vi "AlazarSampling.vi"(9 "Time Out (s)":dbl, 10 "Sampling (Hz)":dbl, 11 "DeviceIn":i32) -> (0 "Return Code":u32, 3 "DeviceOut":i32)   [LabVIEW 2022 SP3]
doc: "_____AlazarTech, Scope_____\n\nConfigure the capture clock circuitry."
uses:
  C:/AlazarTech/ATS-VI/6.2.0/ATS_ctl/Device_Ctrl.ctl
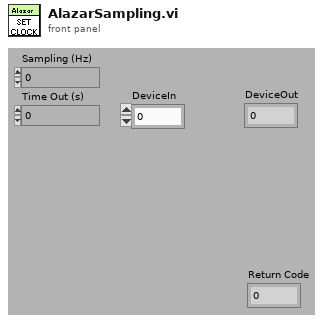
[diagram p1: front panel]
types:
  T1 = typedef "Device_Ctrl.ctl" = enum16{"Status", "About", "Arm", "ForceTrig", "Abort", "Initialize", "Init (NoPreset)", "Info", "Close", "Calibrate", "SetManually", "LED_ON", "LED_OFF"}
  T2 = typedef "Device_Info.ctl" = cluster{"Handle":u32, "Board":string, "CPLD":string, "MemorySize":u32, "SampleSize":u8, "ID":i32, "High_Memory":bool, "Chan/Board":u8}
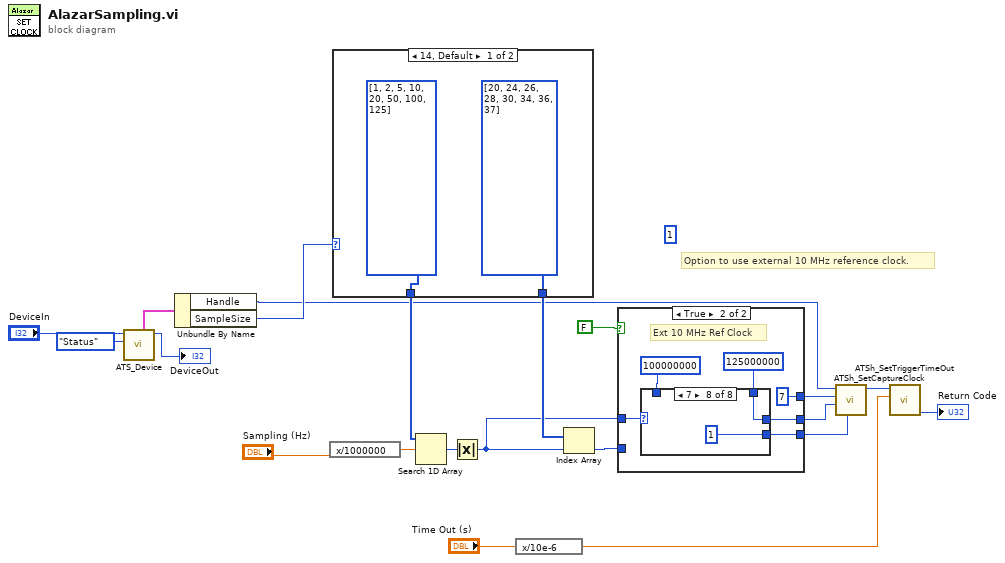
[diagram p0: block diagram]
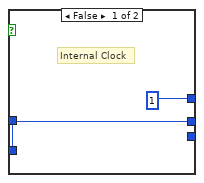
[diagram p2: hidden frame]
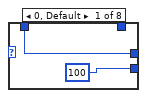
[diagram p3: hidden frame]
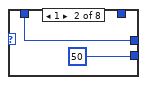
[diagram p4: hidden frame]
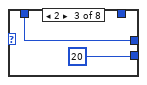
[diagram p5: hidden frame]
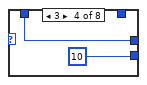
[diagram p6: hidden frame]
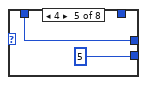
[diagram p7: hidden frame]
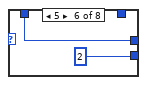
[diagram p8: hidden frame]
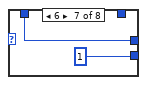
[diagram p9: hidden frame]
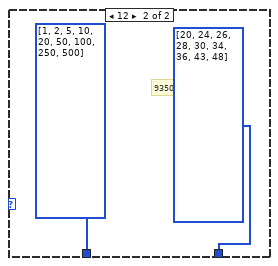
[diagram p10: hidden frame]
diagram:
  (unwired) u32 1 ("Decimation")
  # "Option to use external 10 MHz reference clock."
  n1 = call "ATS_Device.vi"("DevCtrl"=Device_Ctrl."Status", "DeviceIn"="DeviceIn") -> ("DeviceOut"=→"DeviceOut":i32, "DevInfo"=w16:T2)  [unwired: 3 in, 5 out]
  n2 = Unbundle By Name(w16) -> ("Handle"=w11:u32, "SampleSize"=w12:u8)
  n3 = expression code="x/1000000"("Sampling (Hz)") -> (w21:dbl)
  n4 = case shown="14, Default" w12 {
    tunnel: [i32[] [1, 2, 5, 10, 20, 50, 100, 125] i32[] [1, 2, 5, 10, 20, 50, 100, 250, 500]] -> w20
    tunnel: [i32[] [20, 24, 26, 28, 30, 34, 36, 37] i32[] [20, 24, 26, 28, 30, 34, 36, 43, 48]] -> w19
    frame 14, Default {
      # "9440"
    }
    frame 12 {
      # "9350"
    }
  }
  n5 = Search 1D Array(1D array=w20, element=w21) -> (index of element=w18:i32)  [unwired: 1 in]
  n6 = Absolute Value(x=w18) -> (abs(x)=w2:i32)
  n7 = expression code="x/10e-6"("Time Out (s)") -> (w13:dbl)
  n8 = Index Array(array=w19, index=w2) -> (element=w5:i32)
  n9 = case shown="True" FALSE {
    tunnel: [u32 1 ("Source") u32 7 ("Source")] -> w6
    tunnel: w5 -> [w26 _]
    tunnel: [w26 w31] -> w4
    tunnel: w2 -> [_ w32]
    tunnel: [_ w29] -> w1
    frame False {
      # "Internal Clock"
    }
    frame True {
      # "Ext 10 MHz Ref Clock"
      n10 = case shown="7" w32 {
        tunnel: [w35 w37 w39 w41 w43 w45 w47 w49] -> w31
        tunnel: u32 125000000 ("Rate") -> [_ _ _ _ _ _ _ w49]
        tunnel: [u32 100 ("Source") u32 50 ("Source") u32 20 ("Source") u32 10 ("Source") u32 5 ("Source") u32 2 ("Source") u32 1 ("Source") u32 1 ("Source")] -> w29
        tunnel: u32 100000000 ("Rate") -> [w35 w37 w39 w41 w43 w45 w47 _]
        frame 0, Default {
        }
        frame 1 {
        }
        frame 2 {
        }
        frame 3 {
        }
        frame 4 {
        }
        frame 5 {
        }
        frame 6 {
        }
        frame 7 {
        }
      }
    }
  }
  n11 = call "ATSh_SetCaptureClock.vi"("Decimation"=w1, "Rate"=w4, "Source"=w6, "Handle"=w11) -> ("Handle_Out"=w10:u32)  [unwired: 6 in, 1 out]
  n12 = call "ATSh_SetTriggerTimeOut.vi"("TimeoutCount"=w13, "Handle"=w10) -> ("Return Code"=→"Return Code":u32)  [unwired: 8 in, 1 out]
